vi "Library Owning Palette.vi"(0 "Destination":path) -> (1 "Name":string, 2 "URL":string)   [LabVIEW 2018, in "Scripts.lvlib"]
uses:
  Scripts.lvlib
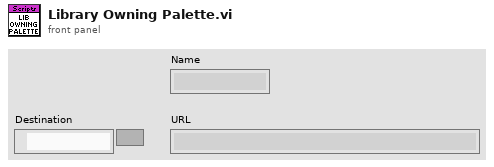
[diagram p1: front panel]
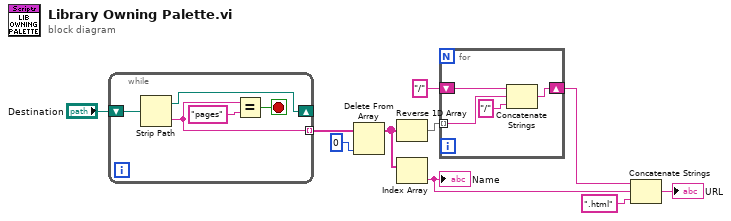
[diagram p0: block diagram]
diagram:
  n1 = while {
    shift-right: [w12] -> _
    shift-left: "Destination" -> [w15]
    tunnel: [w11] -> w3 mode=indexing
    stop <- w13 stop-if-true
    n2 = Strip Path(path=w15) -> (stripped path=w12:path, name=w11:string)
    n3 = Equal?(x=w11, y="pages") -> (x = y?=w13:bool)
  }
  n4 = Delete From Array(array=w3, index=0) -> (array with subset deleted=w2:string[])  [unwired: 1 in, 1 out]
  n5 = Reverse 1D Array(array=w2) -> (reversed array=w5:string[])
  n6 = Index Array(array=w2) -> (element=w10:string)  [unwired: 1 in]
  "Name" <- w10
  n7 = for {
    tunnel: w5 -> [w18] mode=indexing
    shift-right: [w16] -> w7
    shift-left: "/" -> [w19]
    n8 = Concatenate Strings(w19, w18, "/") -> (w16:string)
  }
  n9 = Concatenate Strings(w7, w10, ".html" ("string")) -> (→"URL":string)
